vi "Create.vi"(8 "error in (no error)":errorcluster, 10 "Report":refnum<class "Report Interface.lvclass">) -> (0 "error out":errorcluster, 3 "Report Generator Out":refnum<class "Report Generator.lvclass">)   [LabVIEW 2020, in "Reports.lvlib" / "Report Generator.lvclass"]
uses:
  Report Generator.lvclass
  Framework/Report Interface/Report Interface.lvclass
  Report Generator.lvclass/Report Generator.ctl
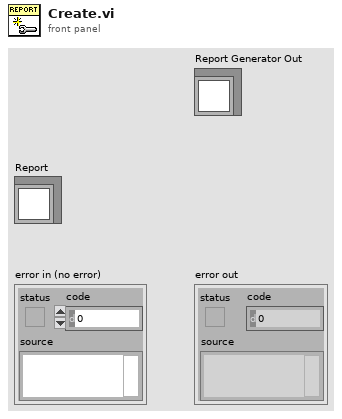
[diagram p1: front panel]
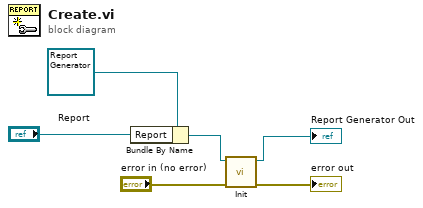
[diagram p0: block diagram]
diagram:
  n1 = Bundle By Name(cluster=refnum<class "Report Generator.lvclass"> refnum ("Report Generator in"), "Report"="Report") -> (w4:refnum<class "Report Generator.lvclass">)
  n2 = call-dynamic "Init.vi"("error in (no error)"="error in (no error)", "Report Generator In"=w4) -> ("error out"=→"error out":errorcluster, "Report Generator Out"=→"Report Generator Out":refnum<class "Report Generator.lvclass">)  [unwired: 8 in]
